vi "Format Headers.vi"(8 "error in (no error)":errorcluster, 9 "Column.Headers":bool, 10 "Row.Headers":bool, 11 "xwpfTable in":refnum<class "xwpfTable.lvclass">) -> (0 "error out":errorcluster, 3 "xwpfTable out":refnum<class "xwpfTable.lvclass">)   [LabVIEW 2017, in "Word_Specific.lvlib" / "xwpfTable.lvclass"]
uses:
  xwpfTable.lvclass
  xwpfTable.lvclass/xwpfTable.ctl
  Styles/Heading 3/Heading 3.lvclass
  C:/Users/Neo/Desktop/Dev_Tools_BR/LabVIEW_NPOI/src/Styles/Style/Style.lvclass
  xwpfParagraph/xwpfParagraph.lvclass
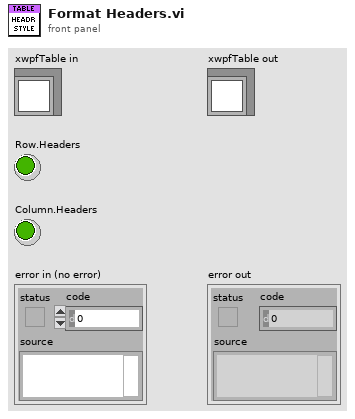
[diagram p1: front panel]
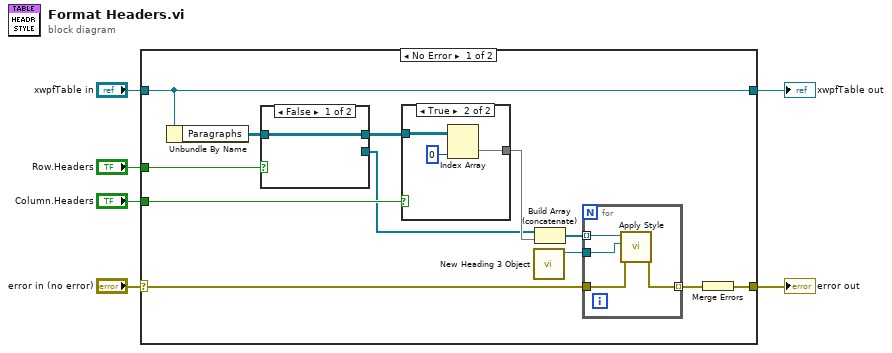
[diagram p0: block diagram]
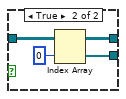
[diagram p3: hidden frame]
diagram:
  n1 = case shown="No Error" "error in (no error)" {
    selector: "error in (no error)" -> [w10 w31]
    tunnel: [w8 w31] -> w5
    tunnel: [w18 w30] -> w3
    tunnel: "xwpfTable in" -> [w18 w30]
    tunnel: "Row.Headers" -> [w16 _]
    tunnel: "Column.Headers" -> [w14 _]
    frame No Error {
      n2 = Unbundle By Name(w18) -> ("Paragraphs"=w17:refnum<class "xwpfParagraph.lvclass">[][])
      n3 = case shown="False" w16 {
        tunnel: w17 -> [w26 w27]
        tunnel: [_ w28] -> w12
        tunnel: [w26 w27] -> w15
        frame False {
        }
        frame True {
          n4 = Index Array(array=w27, index (row)=0) -> (element=w28:refnum<class "xwpfParagraph.lvclass">[])  [unwired: 1 in]
        }
      }
      n5 = case shown="True" w14 {
        tunnel: w15 -> [_ w24]
        tunnel: [_ w25] -> w13
        frame False {
        }
        frame True {
          n6 = Index Array(array=w24, index (col)=0 ("index (row)")) -> (element=w25:refnum<class "xwpfParagraph.lvclass">[])  [unwired: 1 in]
        }
      }
      n7 = call "New Heading 3 Object.vi"() -> ("Heading 3 out"=w7:refnum<class "Heading 3.lvclass">)  [unwired: 10 in, 1 out]
      n8 = Build Array (concatenate)(w12, w13) -> (w11:refnum<class "xwpfParagraph.lvclass">[])
      n9 = for {
        tunnel: w11 -> [w22] mode=indexing
        tunnel: [w21] -> w9 mode=indexing
        tunnel: w10 -> [w20]
        tunnel: w7 -> [w19]
        n10 = call "Apply Style.vi"("error in (no error)"=w20, "Headers.Style"=w19, "xwpfParagraph in"=w22) -> ("error out"=w21:errorcluster)  [unwired: 7 in, 1 out]
      }
      n11 = Merge Errors(w9) -> (w8:errorcluster)
    }
    frame Error {
    }
  }
  "error out" <- w5
  "xwpfTable out" <- w3
